vi "Greater Than.vi"(10 "Numeric 5":dbl, 11 "Numeric 6":dbl) -> (3 "Numeric 7":dbl)   [LabVIEW 2016]
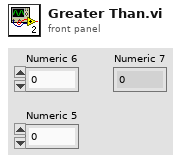
[diagram p1: front panel]
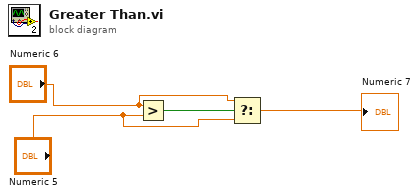
[diagram p0: block diagram]
diagram:
  n1 = Greater?(x="Numeric 6", y="Numeric 5") -> (0:w1:bool)
  n2 = Select(t="Numeric 6", s=w1, f="Numeric 5") -> (s? t:f=→"Numeric 7":dbl)
